vi "Facade 1.vi"(0 "Data In":T20, 2 "Display State In":T18, 3 "Container State":T19) -> (6 "Data Out":T20, 7 "Display State Out":T18, 8 "Action":T17)   [LabVIEW 2020, in "xMessageType.xctl"]
uses:
  xMessageType.xctl
  Data 1.ctl
  MessageBase/MessageBase.lvclass
  <vilib>/_xctls/Container State.ctl
  State 1.ctl
  <vilib>/_xctls/Action.ctl
  MessageType.ctl
  Time/Time.Parameters.ctl
  AddOrder/AddOrderLong.Parameters.ctl
  AddOrder/AddOrderShort.Parameters.ctl
  AddOrder/AddOrderExpanded.Parameters.ctl
  OrderExecuted/OrderExecuted.Parameters.ctl
  OrderExecuted/OrderExecutedAtPriceSize.Parameters.ctl
  ReduceSize/ReduceSizeLong.Parameters.ctl
  ReduceSize/ReduceSizeShort.Parameters.ctl
  ModifyOrder/ModifyOrderLong.Parameters.ctl
  ModifyOrder/ModifyOrderShort.Parameters.ctl
  DeleteOrder/DeleteOrder.Parameters.ctl
  Trade/TradeLong.Parameters.ctl
  Trade/TradeShort.Parameters.ctl
  Trade/TradeExpanded.Parameters.ctl
  AddOrder/AddOrderShort.lvclass
  C:/work/fpganow/cboe_pitch_lv_fpga/cboe_pitch/host/bats.parser/pitch/MessageBase/MessageBase.lvclass
  AddOrder/AddOrderExpanded.lvclass
  OrderExecuted/OrderExecuted.lvclass
  OrderExecuted/OrderExecutedAtPriceSize.lvclass
  ReduceSize/ReduceSizeLong.lvclass
  ReduceSize/ReduceSizeShort.lvclass
  ModifyOrder/ModifyOrderLong.lvclass
  ModifyOrder/ModifyOrderShort.lvclass
  DeleteOrder/DeleteOrder.lvclass
  Trade/TradeLong.lvclass
  Trade/TradeShort.lvclass
  Trade/TradeExpanded.lvclass
  <vilib>/_xctls/XControlSupport.lvlib
  AddOrder/AddOrderLong.lvclass
  Time/Time.lvclass
panel:
  out "data.change":string
  in  "MessageTypeTab":T1(tab)
  in  "Time.Parameters":T2
  in  "AddOrderLong.Parameters":T3
  in  "AddOrderShort.Parameters":T4
  in  "AddOrderExpanded.Parameters":T5
  in  "OrderExecuted.Parameters":T6
  in  "OrderExecutedAtPriceSize.Parameters":T7
  in  "ReduceSizeLong.Parameters":T8
  in  "ReduceSizeShort.Parameters":T9
  in  "ModifyOrderLong.Parameters":T10
  in  "ModifyOrderShort.Parameters":T11
  in  "DeleteOrder.Parameters":T12
  in  "TradeLong.Parameters":T13
  in  "TradeShort.Parameters":T14
  in  "TradeExpanded.Parameters":T15
  in  "Message Type":T16
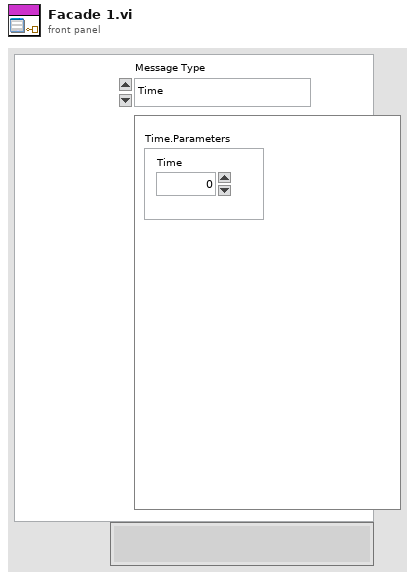
[diagram p1: front panel]
types:
  T1 = enum32{"Time", "AddOrderLong", "AddOrderShort", "AddOrderExpanded", "OrderExecuted", "OrderExecutedAtPriceSize", "ReduceSizeLong", "ReduceSizeShort", "ModifyOrderLong", "ModifyOrderShort", "DeleteOrder", "TradeLong", "TradeShort", "TradeExpanded"}
  T2 = typedef "Time.lvclass/Time.Parameters.ctl" = cluster{"Time":u32}
  T3 = typedef "AddOrderLong.lvclass/AddOrderLong.Parameters.ctl" = cluster{"Time Offset":u32, "Order Id":string, "Quantity":u32, "Symbol":string, "Side Indicator":string, "Price":dbl}
  T4 = typedef "AddOrderShort.lvclass/AddOrderShort.Parameters.ctl" = cluster{"Time Offset":u32, "Order Id":string, "Quantity":u32, "Symbol":string, "Side Indicator":string, "Price":dbl}
  T5 = typedef "AddOrderExpanded.lvclass/AddOrderExpanded.Parameters.ctl" = cluster{"Time Offset":u32, "Order Id":string, "Quantity":u32, "Symbol":string, "Side Indicator":string, "Price":dbl, "Participant Id":string, "Customer Indicator":string}
  T6 = typedef "OrderExecuted.lvclass/OrderExecuted.Parameters.ctl" = cluster{"Time Offset":u32, "Order Id":string, "Executed Quantity":u32, "Execution Id":string}
  T7 = typedef "OrderExecutedAtPriceSize.lvclass/OrderExecutedAtPriceSize.Parameters.ctl" = cluster{"Time Offset":u32, "Order Id":string, "Executed Quantity":u32, "Execution Id":string, "Remaining Quantity":u32, "Price":dbl}
  T8 = typedef "ReduceSizeLong.lvclass/ReduceSizeLong.Parameters.ctl" = cluster{"Time Offset":u32, "Order Id":string, "Canceled Quantity":u32}
  T9 = typedef "ReduceSizeShort.lvclass/ReduceSizeShort.Parameters.ctl" = cluster{"Time Offset":u32, "Order Id":string, "Canceled Quantity":u16}
  T10 = typedef "ModifyOrderLong.lvclass/ModifyOrderLong.Parameters.ctl" = cluster{"Time Offset":u32, "Order Id":string, "Quantity":u32, "Price":dbl, "Modify Flags":u8}
  T11 = typedef "ModifyOrderShort.lvclass/ModifyOrderShort.Parameters.ctl" = cluster{"Time Offset":u32, "Order Id":string, "Quantity":u32, "Price":u16, "Modify Flags":u8}
  T12 = typedef "DeleteOrder.lvclass/DeleteOrder.Parameters.ctl" = cluster{"Time Offset":u32, "Order Id":string}
  T13 = typedef "TradeLong.lvclass/TradeLong.Parameters.ctl" = cluster{"Time Offset":u32, "Order Id":string, "Execution Id":string, "Quantity":u32, "Price":dbl, "Side Indicator":string, "Symbol":string}
  T14 = typedef "TradeShort.lvclass/TradeShort.Parameters.ctl" = cluster{"Time Offset":u32, "Order Id":string, "Execution Id":string, "Quantity":u32, "Price":dbl, "Side Indicator":string, "Symbol":string}
  T15 = typedef "TradeExpanded.lvclass/TradeExpanded.Parameters.ctl" = cluster{"Time Offset":u32, "Order Id":string, "Side Indicator":string, "Quantity":u32, "Symbol":string, "Price":dbl, "Execution Id":string}
  T16 = typedef "MessageType.ctl" = enum16{"Time", "AddOrderLong", "AddOrderShort", "AddOrderExpanded", "OrderExecuted", "OrderExecutedAtPriceSize", "ReduceSizeLong", "ReduceSizeShort", "ModifyOrderLong", "ModifyOrderShort", "DeleteOrder", "TradeLong", "TradeShort", "TradeExpanded"}
  T17 = typedef "XControlSupport.lvlib/Action.ctl" = cluster{"Data Changed?":bool, "State Changed?":bool, "Action Name":string}
  T18 = typedef "xMessageType.xctl/State 1.ctl" = cluster{"state.string":string, "state.number":u32, "MessageBase.lvclass":refnum<class "MessageBase.lvclass">}
  T19 = typedef "XControlSupport.lvlib/Container State.ctl" = cluster{"Indicator?":bool, "Run Mode?":bool, " Refnum":refnum<vi>}
  T20 = typedef "xMessageType.xctl/Data 1.ctl" = cluster{"MessageBase.lvclass":refnum<class "MessageBase.lvclass">, "data.string":string}
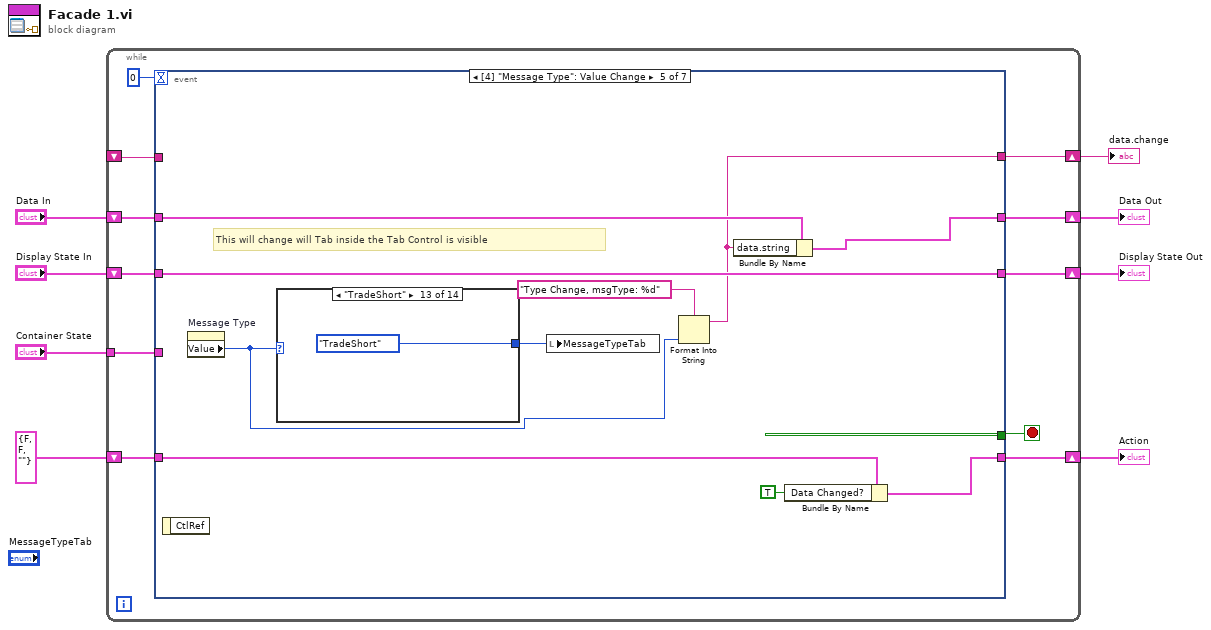
[diagram p0: block diagram]
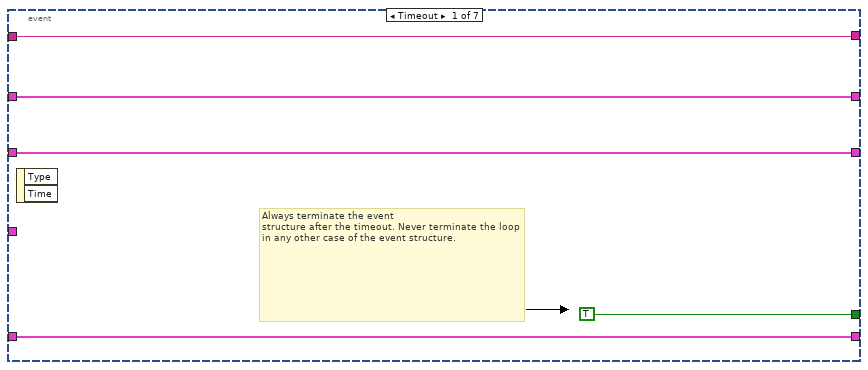
[diagram p2: hidden frame]
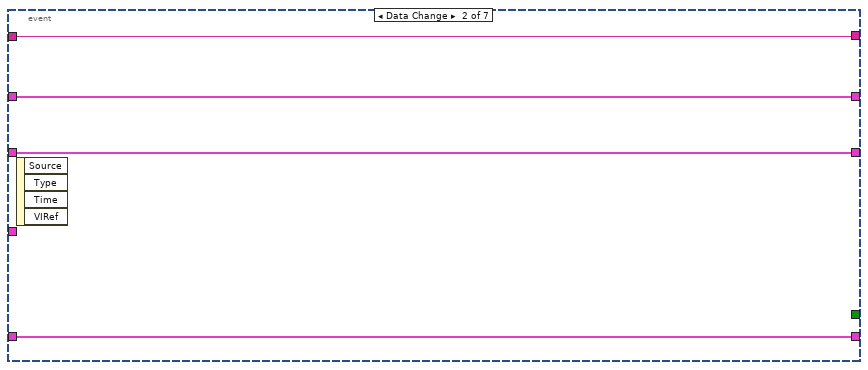
[diagram p3: hidden frame]
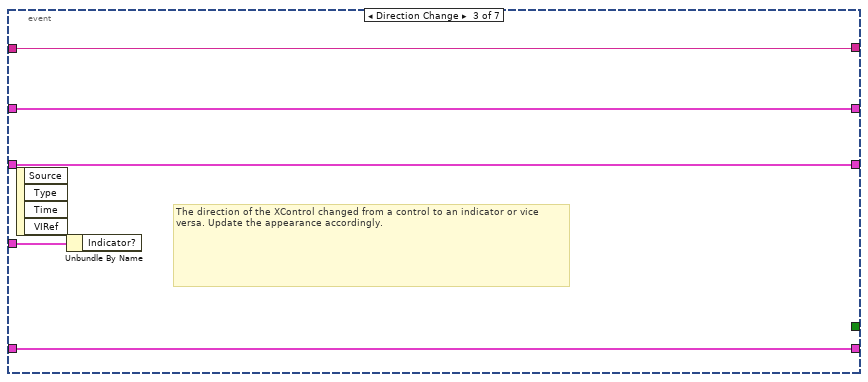
[diagram p4: hidden frame]
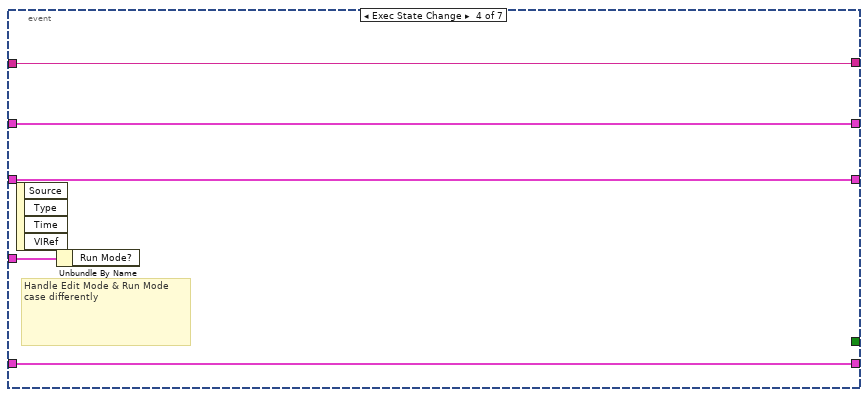
[diagram p5: hidden frame]
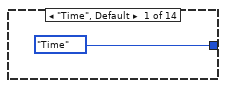
[diagram p6: hidden frame]
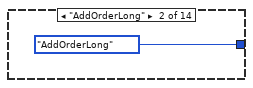
[diagram p7: hidden frame]
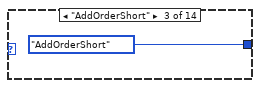
[diagram p8: hidden frame]
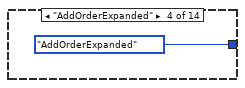
[diagram p9: hidden frame]
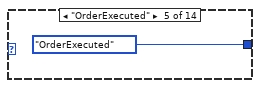
[diagram p10: hidden frame]
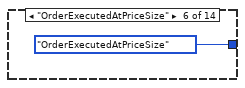
[diagram p11: hidden frame]
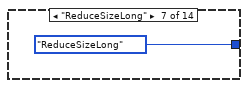
[diagram p12: hidden frame]
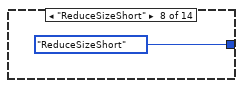
[diagram p13: hidden frame]
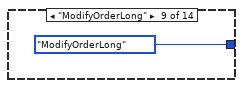
[diagram p14: hidden frame]
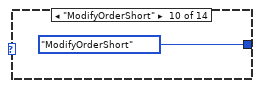
[diagram p15: hidden frame]
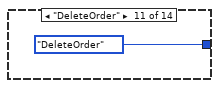
[diagram p16: hidden frame]
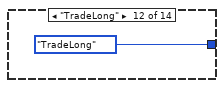
[diagram p17: hidden frame]
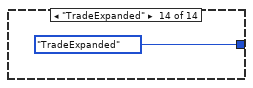
[diagram p18: hidden frame]
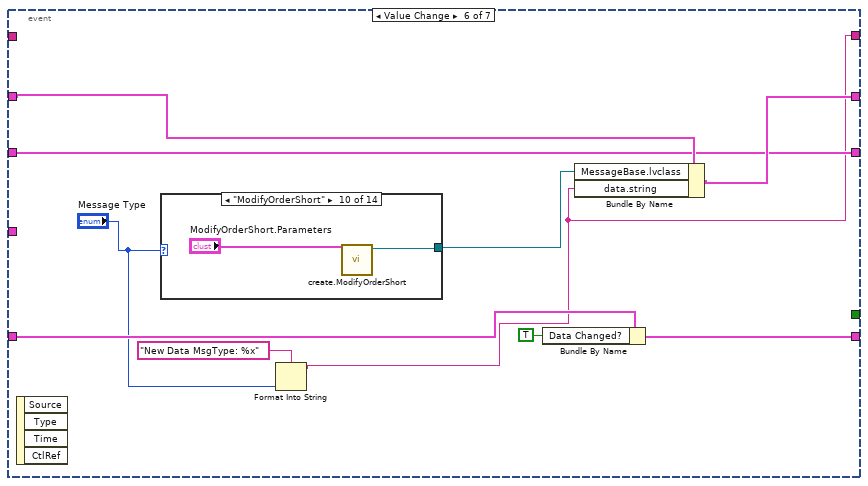
[diagram p19: hidden frame]
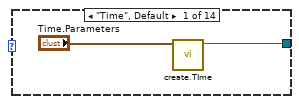
[diagram p20: hidden frame]
diagram:
  n1 = while {
    shift-right: [w18] -> w5
    shift-left: "Display State In" -> [w19]
    tunnel: "Container State" -> [w15]
    shift-right: [w13] -> w8
    shift-left: "Data In" -> [w14]
    shift-right: [w11] -> w3
    shift-left: T17 {"Data Changed?"=FALSE, "State Changed?"=FALSE, "Action Name"=""} ("Action") -> [w12]
    shift-right: [w10] -> w1
    shift-left: _ -> [w9]
    stop <- w17 stop-if-true
    n2 = event shown="[4] \"Message Type\": Value Change" {
      selector: _ -> [_ _ _ _ _ _ _]
      dyn-events: _ -> [_ _ _ _ _ _ _]
      timeout: 0 -> [_ _ _ _ _ _ _]
      tunnel: w19 -> [w22 w27 w32 w37 w47 w66 w104]
      tunnel: [w22 w27 w32 w37 w47 w66 w104] -> w18
      tunnel: [TRUE _ _ _ _ _ _] -> w17
      tunnel: w15 -> [_ _ w33 w38 _ _ _]
      tunnel: w14 -> [w21 w26 w31 w35 w46 w67 w103]
      tunnel: [w21 w26 w31 w35 w45 w68 w103] -> w13
      tunnel: [w23 w28 w30 w36 w41 w69 w102] -> w11
      tunnel: w12 -> [w23 w28 w30 w36 w42 w70 w102]
      tunnel: [w20 w25 w29 w34 w39 w63 w101] -> w10
      tunnel: w9 -> [w20 w25 w29 w34 _ _ w101]
      event Timeout {
        # "Always terminate the event\nstructure after the timeout. Never terminate the loop in any other case of the event structure."
        n3 = event-data() -> ()  [unwired: 1 in, 2 out]
      }
      event Data Change {
        n4 = event-data() -> ()  [unwired: 1 in, 4 out]
      }
      event Direction Change {
        # "The direction of the XControl changed from a control to an indicator or vice versa. Update the appearance accordingly."
        n5 = event-data() -> ()  [unwired: 1 in, 4 out]
        n6 = Unbundle By Name(w33) -> ()  [unwired: 1 out]
      }
      event Exec State Change {
        # "Handle Edit Mode & Run Mode\ncase differently"
        n7 = event-data() -> ()  [unwired: 1 in, 4 out]
        n8 = Unbundle By Name(w38) -> ()  [unwired: 1 out]
      }
      event Value Change {
        # "This will change will Tab inside the Tab Control is visible"
        n9 = event-data() -> ()  [unwired: 1 in, 1 out]
        n10 = property on="Message Type" class="Enum (strict)"() -> ("Value"=w44:T16)  [unwired: 2 in, 2 out]
        n11 = case shown="\"TradeShort\"" w44 {
          tunnel: [T1."Time" ("MessageTypeTab") T1."AddOrderLong" ("MessageTypeTab") T1."AddOrderShort" ("MessageTypeTab") T1."AddOrderExpanded" ("MessageTypeTab") T1."OrderExecuted" ("MessageTypeTab") T1."OrderExecutedAtPriceSize" ("MessageTypeTab") T1."ReduceSizeLong" ("MessageTypeTab") T1."ReduceSizeShort" ("MessageTypeTab") T1."ModifyOrderLong" ("MessageTypeTab") T1."ModifyOrderShort" ("MessageTypeTab") T1."DeleteOrder" ("MessageTypeTab") T1."TradeLong" ("MessageTypeTab") T1."TradeShort" ("MessageTypeTab") T1."TradeExpanded" ("MessageTypeTab")] -> w48
          frame "Time", Default {
          }
          frame "AddOrderLong" {
          }
          frame "AddOrderShort" {
          }
          frame "AddOrderExpanded" {
          }
          frame "OrderExecuted" {
          }
          frame "OrderExecutedAtPriceSize" {
          }
          frame "ReduceSizeLong" {
          }
          frame "ReduceSizeShort" {
          }
          frame "ModifyOrderLong" {
          }
          frame "ModifyOrderShort" {
          }
          frame "DeleteOrder" {
          }
          frame "TradeLong" {
          }
          frame "TradeShort" {
          }
          frame "TradeExpanded" {
          }
        }
        n12 = local write "MessageTypeTab"(w48) -> ()
        n13 = Format Into String(format string="Type Change, msgType: %d", w44) -> (resulting string=w39:string)  [unwired: 2 in, 1 out]
        n14 = Bundle By Name(cluster=w46, "data.string"=w39) -> (w45:T20)
        n15 = Bundle By Name(cluster=w42, "Data Changed?"=TRUE) -> (w41:T17)
      }
      event Value Change {
        n16 = event-data() -> ()  [unwired: 1 in, 4 out]
        n17 = case shown="\"ModifyOrderShort\"" "Message Type" {
          tunnel: [w74 w76 w78 w80 w81 w83 w86 w87 w90 w91 w93 w95 w97 w99] -> w71
          frame "Time", Default {
            n18 = call "create.TIme.vi"("Time.Parameters"="Time.Parameters") -> ("MessageBase out"=w74:refnum<class "MessageBase.lvclass">)  [unwired: 8 in, 2 out]
          }
          frame "AddOrderLong" {
            n19 = call "create.AddOrderLong.vi"("AddOrderLong.Parameters"="AddOrderLong.Parameters") -> ("MessageBase out"=w76:refnum<class "MessageBase.lvclass">)  [unwired: 9 in, 1 out]
          }
          frame "AddOrderShort" {
            n20 = call "create.AddOrderShort.vi"("AddOrderShort.Parameters"="AddOrderShort.Parameters") -> ("MessageBase out"=w78:refnum<class "AddOrderShort.lvclass">)  [unwired: 9 in, 1 out]
          }
          frame "AddOrderExpanded" {
            n21 = call "create.AddOrderExpanded.vi"("AddOrderExpanded.Parameters"="AddOrderExpanded.Parameters") -> ("MessageBase out"=w80:refnum<class "AddOrderExpanded.lvclass">)  [unwired: 9 in, 1 out]
          }
          frame "OrderExecuted" {
            n22 = call "create.OrderExecuted.vi"("OrderExecuted.Parameters"="OrderExecuted.Parameters") -> ("MessageBase out"=w81:refnum<class "OrderExecuted.lvclass">)  [unwired: 9 in, 1 out]
          }
          frame "OrderExecutedAtPriceSize" {
            n23 = call "create.OrderExecutedAtPriceSize.vi"("OrderExecutedAtPriceSize.Parameters"="OrderExecutedAtPriceSize.Parameters") -> ("MessageBase out"=w83:refnum<class "OrderExecutedAtPriceSize.lvclass">)  [unwired: 9 in, 1 out]
          }
          frame "ReduceSizeLong" {
            n24 = call "create.ReduceSizeLong.vi"("ReduceSizeLong.Parameters"="ReduceSizeLong.Parameters") -> ("ReduceSizeLong"=w86:refnum<class "ReduceSizeLong.lvclass">)  [unwired: 8 in, 2 out]
          }
          frame "ReduceSizeShort" {
            n25 = call "create.ReduceSizeShort.vi"("ReduceSizeShort.Parameters"="ReduceSizeShort.Parameters") -> ("MessageBase out"=w87:refnum<class "ReduceSizeShort.lvclass">)  [unwired: 8 in, 2 out]
          }
          frame "ModifyOrderLong" {
            n26 = call "create.ModifyOrderLong.vi"("ModifyOrderLong.Parameters"="ModifyOrderLong.Parameters") -> ("MessageBase out"=w90:refnum<class "ModifyOrderLong.lvclass">)  [unwired: 8 in, 2 out]
          }
          frame "ModifyOrderShort" {
            n27 = call "create.ModifyOrderShort.vi"("ModifyOrderShort.Parameters"="ModifyOrderShort.Parameters") -> ("MessageBase out"=w91:refnum<class "ModifyOrderShort.lvclass">)  [unwired: 8 in, 2 out]
          }
          frame "DeleteOrder" {
            n28 = call "create.DeleteOrder.vi"("DeleteOrder.Parameters"="DeleteOrder.Parameters") -> ("MessageBase out"=w93:refnum<class "DeleteOrder.lvclass">)  [unwired: 8 in, 2 out]
          }
          frame "TradeLong" {
            n29 = call "create.TradeLong.vi"("TradeLong.Parms"="TradeLong.Parameters") -> ("MessageBase out"=w95:refnum<class "TradeLong.lvclass">)  [unwired: 8 in, 2 out]
          }
          frame "TradeShort" {
            n30 = call "create.TradeShort.vi"("TradeShort.Parmeters"="TradeShort.Parameters") -> ("MessageBase out"=w97:refnum<class "TradeShort.lvclass">)  [unwired: 8 in, 2 out]
          }
          frame "TradeExpanded" {
            n31 = call "create.TradeExpanded.vi"("TradeExpanded.Parmeters"="TradeExpanded.Parameters") -> ("MessageBase out"=w99:refnum<class "TradeExpanded.lvclass">)  [unwired: 8 in, 2 out]
          }
        }
        n32 = Format Into String(format string="New Data MsgType: %x", "Message Type") -> (resulting string=w63:string)  [unwired: 2 in, 1 out]
        n33 = Bundle By Name(cluster=w70, "Data Changed?"=TRUE) -> (w69:T17)
        n34 = Bundle By Name(cluster=w67, "MessageBase.lvclass"=w71, "data.string"=w63) -> (w68:T20)
      }
      event Panel Resize {
        n35 = event-data() -> ()  [unwired: 1 in, 1 out]
      }
    }
  }
  "Display State Out" <- w5
  "Data Out" <- w8
  "Action" <- w3
  "data.change" <- w1
